vi "time_sub_frame.vi"(7 "Case select":string, 8 "felharmonikus N":i32=2, 9 "SNR window width [Hz]":dbl=0.4 format="%#_13g", 11 "path to binary file":path) -> (3 "output cluster":T1)   [LabVIEW 2017]
uses:
  <vilib>/Utility/file.llb/Read Delimited Spreadsheet (string).vi
  <vilib>/regexp/Match Regular Expression.xnode
panel:
  out "Array 2":dbl[](array[numeric])
  out "header":T2
  out "impulse szum/time (bigger better)":cluster{"X":dbl, "Y":dbl}[](graph)
  out "X SNR 3 (bigger better)":cluster{"X":dbl, "Y":dbl}[](graph)
  out "X SNR 4":cluster{"X":dbl, "Y":dbl}[](graph)
  out "X SNR":cluster{"X":dbl, "Y":dbl}[](graph)
  out "impulse mean (?)":cluster{"X":dbl, "Y":dbl}[](graph)
  out "impulse sd (?)":cluster{"X":dbl, "Y":dbl}[](graph)
  out "impulse szum (?)":cluster{"X":dbl, "Y":dbl}[](graph)
  out "enable":bool
  out "end":timestamp
  out "start":timestamp
  out "state":string
  out "saved":string
  out "all rows":string[][](array[string])
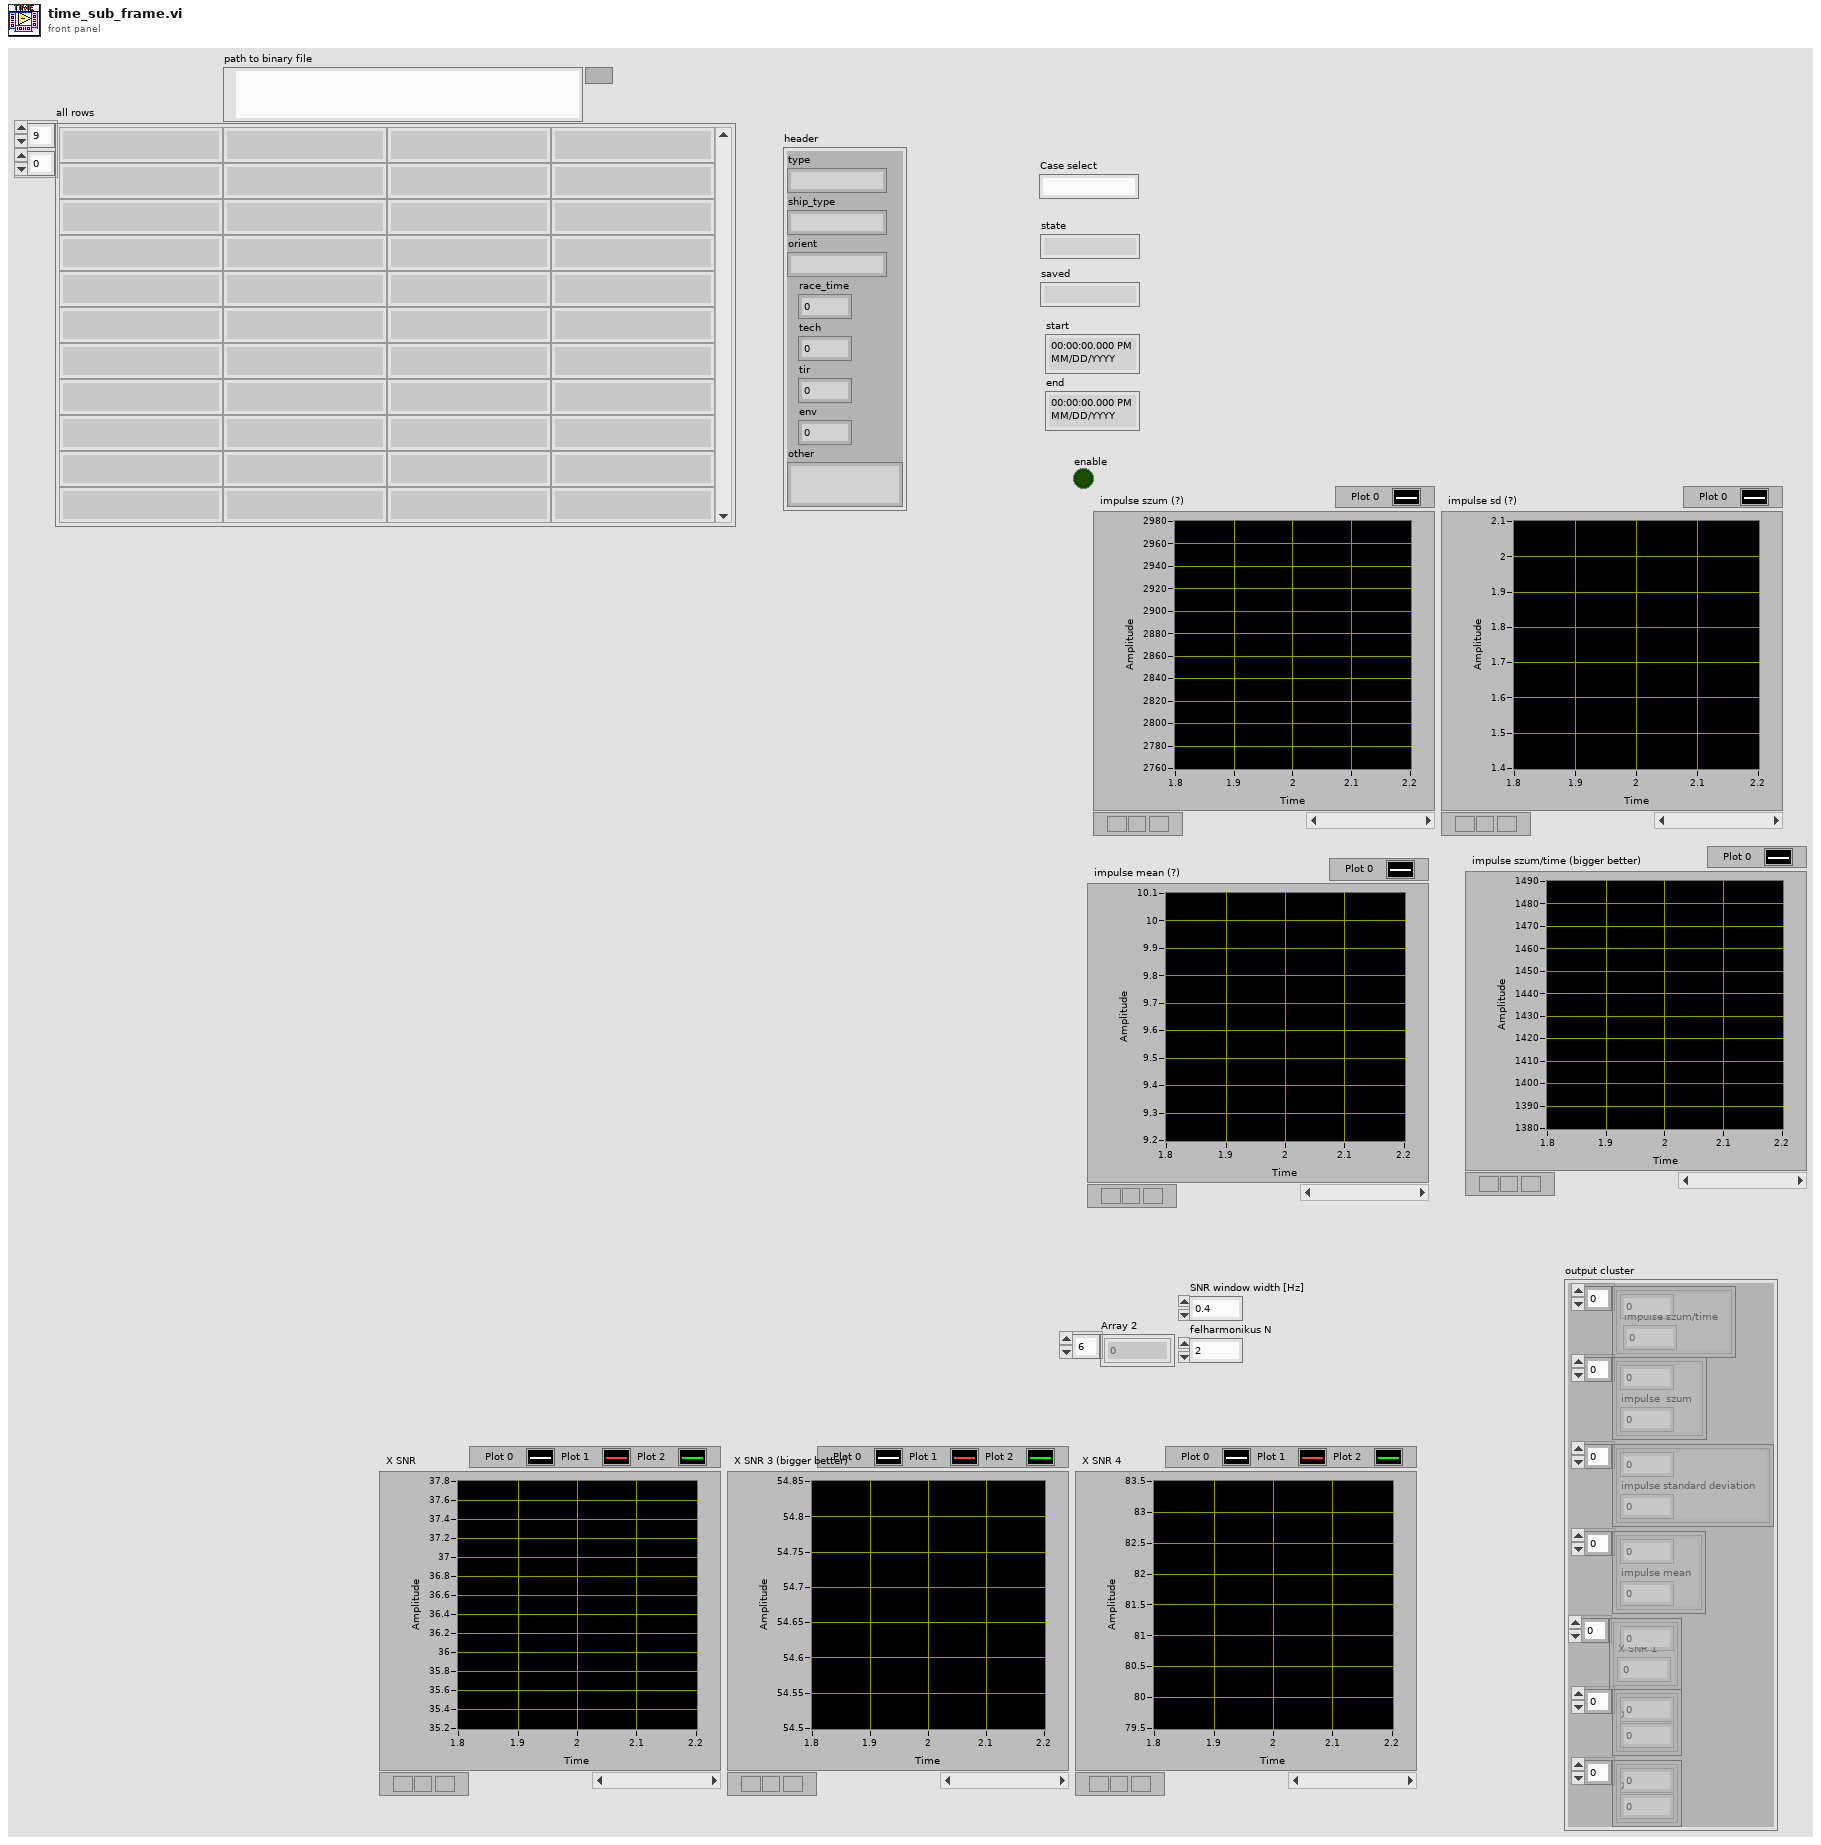
[diagram p1: front panel]
types:
  T1 = cluster{cluster{dbl, "impulse szum/time":dbl}[], cluster{dbl, "impulse  szum":dbl}[], cluster{dbl, "impulse standard deviation":dbl}[], cluster{dbl, "impulse mean":dbl}[], cluster{dbl, "X SNR 1":dbl}[], cluster{dbl, "X SNR 2":dbl}[], cluster{dbl, "X SNR 3":dbl}[]}
  T2 = cluster{"type":string, "ship_type":string, "orient":string, "race_time":dbl, "tech":dbl, "tir":dbl, "env":dbl, "other":string}
  T3 = cluster{cluster{dbl, "impulse szum/time":dbl}[], cluster{dbl, "impulse  szum":dbl}[], cluster{dbl, "impulse standard deviation":dbl}[], cluster{dbl, "impulse mean":dbl}[], cluster{dbl, dbl}[], cluster{dbl, dbl}[], cluster{dbl, dbl}[]}
  T4 = cluster{"path to binary file":path, "Start Cursor":timestamp, "Sec":dbl, "crossing level":dbl, "threshold":dbl, "avg window size":i32, "peak detect width":i32, "invert":bool, "SNR window width [Hz]":dbl, "felharmonikus N":i32, "End cursor":timestamp}
  T5 = cluster{"Átlag Csapásszám [stroke/m]":dbl, "mean of peaks":dbl, "impulse standard deviation":dbl, "impulse  szum":dbl, "standard deviation of peaks":dbl, "impulse mean":dbl, "X axis SNR mean":dbl, "X axis SNR standard deviation":dbl, "Y axis SNR standard deviation":dbl, "Y axis SNR mean":dbl, "resultant SNR standard deviation":dbl, "resultant SNR mean":dbl, "Z axis SNR standard deviation":dbl, "Z axis SNR mean":dbl, "impulse szum/mean":dbl}
  T6 = cluster{cluster{dbl, dbl}[], cluster{dbl, "impulse  szum":dbl}[], cluster{dbl, "impulse standard deviation":dbl}[], cluster{dbl, "impulse mean":dbl}[], cluster{dbl, dbl}[], cluster{dbl, dbl}[], cluster{dbl, dbl}[]}
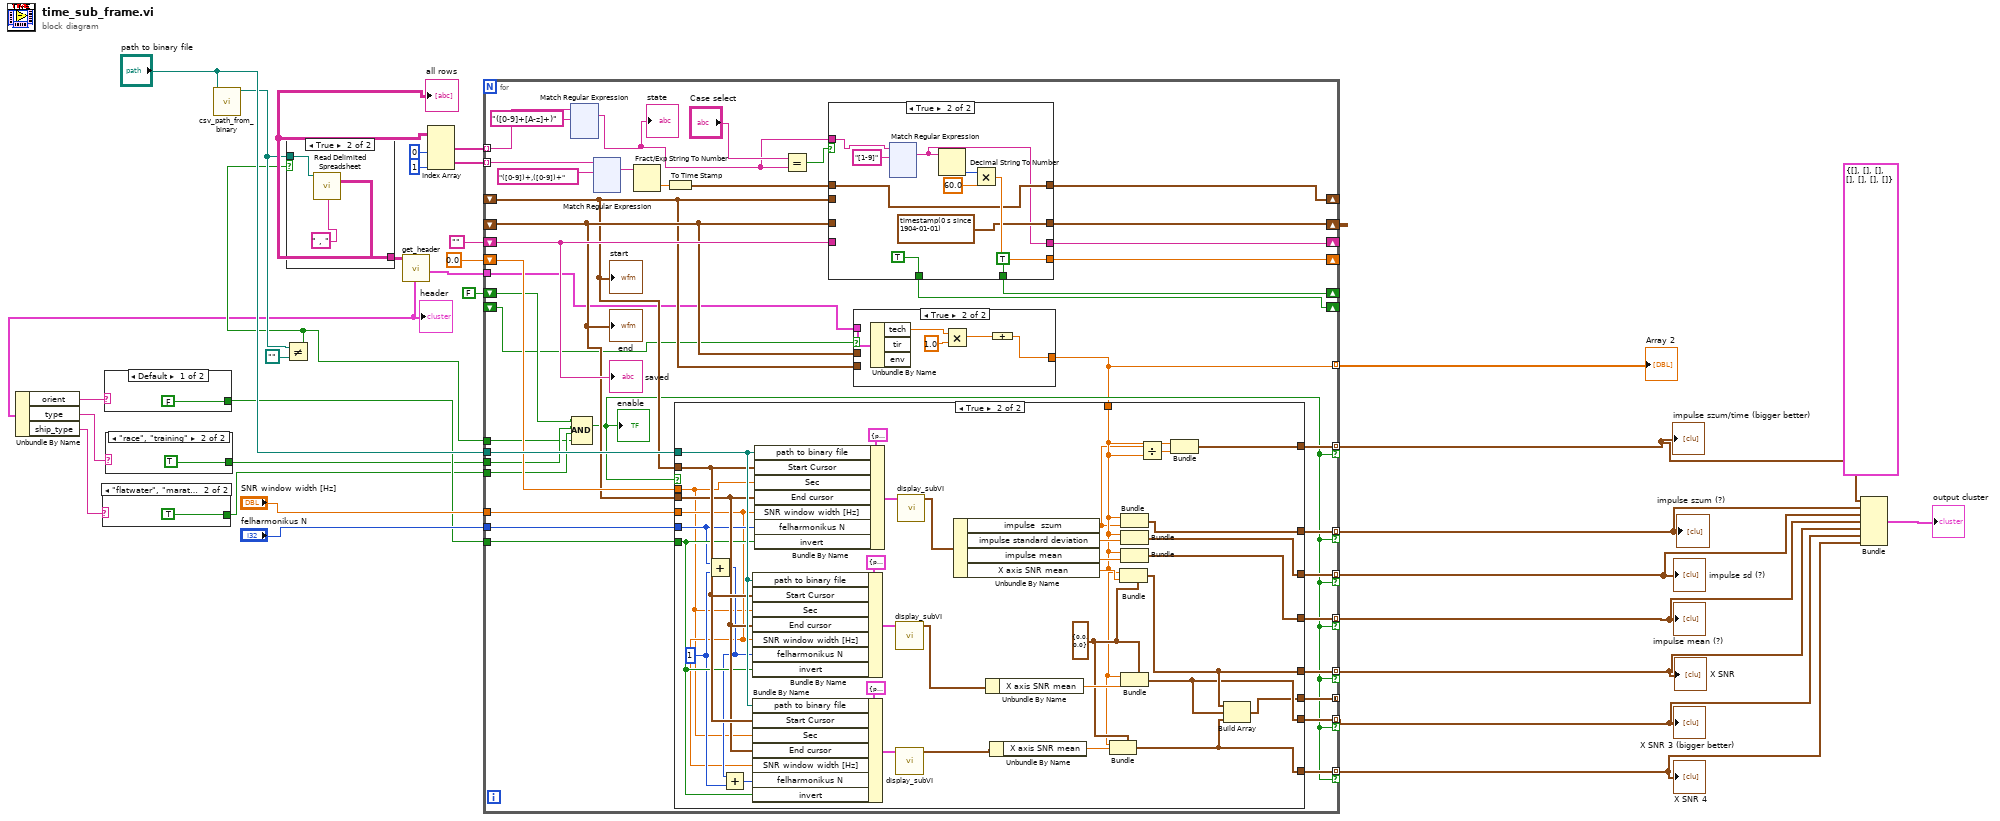
[diagram p0: block diagram]
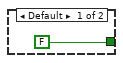
[diagram p3: hidden frame]
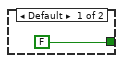
[diagram p4: hidden frame]
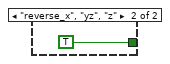
[diagram p5: hidden frame]
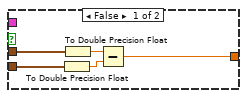
[diagram p6: hidden frame]
diagram:
  (unwired) T3 {[], [], [], [], [], [], []} ("output cluster")
  n1 = call "csv_path_from_binary.vi"("path to binary file"="path to binary file") -> ("path to spec. ext."=w5:path)  [unwired: 10 in]
  n2 = Not Equal?(x=w5, y=path "") -> (x != y?=w4:bool)
  n3 = case shown="True" w4 {
    tunnel: [_ w32] -> w6
    tunnel: w5 -> [_ w31]
    frame False {
    }
    frame True {
      n4 = call-poly <vilib>:"Read Delimited Spreadsheet.vi"("file path (dialog if empty)"=w31, "delimiter (\\t)"=" , " ("delimiter (\\t)")) -> ("all rows"=w32:string[][])  [unwired: 8 in, 5 out]
    }
  }
  "all rows" <- w6
  n5 = call "get_header.vi"("all rows"=w6) -> ("header"=w2:T2)  [unwired: 10 in]
  "header" <- w2
  n6 = Unbundle By Name(w2) -> ("orient"=w21:string, "type"=w11:string, "ship_type"=w9:string)
  n7 = case shown="\"flatwater\", \"marathon\"" w9 {
    tunnel: [FALSE TRUE] -> w8
    frame Default {
    }
    frame "flatwater", "marathon" {
    }
  }
  n8 = case shown="Default" w21 {
    tunnel: [FALSE TRUE] -> w20
    frame Default {
    }
    frame "reverse_x", "yz", "z" {
    }
  }
  n9 = case shown="\"race\", \"training\"" w11 {
    tunnel: [FALSE TRUE] -> w10
    frame Default {
    }
    frame "race", "training" {
    }
  }
  n10 = Index Array(array=w6, index (col) #1=0 ("disabled index (col)"), index (col) #2=1 ("index (col)")) -> (element #1=w29:string[], element #2=w30:string[])  [unwired: 2 in]
  n11 = for {
    tunnel: w30 -> [w76] mode=indexing
    tunnel: w29 -> [w71] mode=indexing
    shift-right: [w74] -> _
    shift-left: _ -> [w61]
    shift-right: [w73] -> _
    shift-left: _ -> [w62]
    shift-right: [w72] -> _
    shift-left: "" -> [w69]
    shift-right: [w47] -> _
    shift-left: 0.0 ("Sec") -> [w66]
    shift-right: [w68] -> _
    shift-left: FALSE -> [w51]
    tunnel: "path to binary file" -> [w67]
    tunnel: "SNR window width [Hz]" -> [w65]
    tunnel: "felharmonikus N" -> [w64]
    tunnel: w20 -> [w63]
    tunnel: [w60] -> w18 mode=indexing if=w52
    tunnel: [w59] -> w17 mode=indexing if=w52
    tunnel: [w58] -> w16 mode=indexing if=w52
    tunnel: [w57] -> w15 mode=indexing if=w52
    tunnel: [w56] -> w14 mode=indexing if=w52
    tunnel: [w55] -> w13 mode=indexing if=w52
    tunnel: [w54] -> _ mode=concatenating
    tunnel: [w53] -> w19 mode=indexing if=w52
    tunnel: w10 -> [w50]
    tunnel: w8 -> [w49]
    tunnel: w4 -> [w48]
    tunnel: w2 -> [w46]
    tunnel: [w45] -> w1 mode=indexing
    shift-right: [w44] -> _
    shift-left: _ -> [w43]
    n12 = xnode "Match Regular Expression"("input string"=w71, "regular expression"="([0-9]+[A-z]+)") -> ("whole match"=w41:string)  [unwired: 4 in, 4 out]
    "state" <- w41
    n13 = Compound Arithmetic op=AND(w51, w50, w49, w48) -> (w52:bool)
    "enable" <- w52
    n14 = xnode "Match Regular Expression"("input string"=w76, "regular expression"="([0-9])+,([0-9])+") -> ("whole match"=w78:string)  [unwired: 4 in, 4 out]
    n15 = Fract/Exp String To Number(string=w78) -> (number=w77:dbl)  [unwired: 3 in, 1 out]
    n16 = To Time Stamp(1:w77) -> (0:w75:timestamp)
    n17 = Equal?(x="Case select", y=w41) -> (x = y?=w40:bool)
    n18 = case shown="True" w40 {
      tunnel: [w240 w248] -> w74
      tunnel: w75 -> [_ w248]
      tunnel: [w241 timestamp(0 s since 1904-01-01) ("f")] -> w73
      tunnel: [w242 w244] -> w72
      tunnel: w69 -> [w242 _]
      tunnel: [_ w249] -> w47
      tunnel: w62 -> [w241 _]
      tunnel: w61 -> [w240 _]
      tunnel: [_ TRUE] -> w68
      tunnel: [_ TRUE] -> w44
      tunnel: w41 -> [_ w243]
      frame False {
      }
      frame True {
        n19 = xnode "Match Regular Expression"("input string"=w243, "regular expression"="[1-9]") -> ("whole match"=w244:string)  [unwired: 4 in, 4 out]
        n20 = Decimal String To Number(string=w244) -> (number=w250:i32)  [unwired: 2 in, 1 out]
        n21 = Multiply(x=w250, y=60.0) -> (x*y=w249:dbl)
      }
    }
    n22 = case shown="True" w43 {
      tunnel: w62 -> [w84 _]
      tunnel: w61 -> [w83 _]
      tunnel: [w80 w86] -> w45
      tunnel: w46 -> [_ w89]
      frame False {
        n23 = To Double Precision Float(number=w83) -> (double precision float=w81:dbl)
        n24 = To Double Precision Float(number=w84) -> (double precision float=w82:dbl)
        n25 = Subtract(x=w82, y=w81) -> (x-y=w80:dbl)
      }
      frame True {
        n26 = Unbundle By Name(w89) -> ("tech"=w88:dbl)  [unwired: 2 out]
        n27 = Multiply(x=w88, y=1.0) -> (x*y=w85:dbl)
        n28 = Compound Arithmetic op=ADD(w85) -> (w86:dbl)
      }
    }
    n29 = case shown="True" w52 {
      tunnel: w67 -> [_ w119]
      tunnel: w61 -> [_ w118]
      tunnel: w62 -> [_ w117]
      tunnel: w66 -> [_ w110]
      tunnel: w65 -> [_ w111]
      tunnel: w64 -> [_ w115]
      tunnel: w63 -> [_ w116]
      tunnel: w45 -> [_ w91]
      tunnel: [_ w105] -> w60
      tunnel: [_ w104] -> w59
      tunnel: [_ w103] -> w58
      tunnel: [_ w98] -> w57
      tunnel: [_ w97] -> w56
      tunnel: [_ w96] -> w55
      tunnel: [_ w95] -> w54
      tunnel: [_ w93] -> w53
      frame False {
      }
      frame True {
        w94 = cluster{dbl, dbl} {0.0, 0.0} ("cluster")
        w112 = 1
        n30 = Add(x=w115, y=w112) -> (x+y=w113:i32)
        n31 = Add(x=w113, y=w112) -> (x+y=w114:i32)
        n32 = Bundle By Name(cluster=T4 {"path to binary file"=path "C:/Users/Lenovo/Desktop/szakdoga/data", "Start Cursor"=timestamp(0 s since 1904-01-01), "Sec"=60.0, "crossing level"=0.0, "threshold"=0.35, "avg window size"=5, "peak detect width"=30, "invert"=FALSE, "SNR window width [Hz]"=0.5, "felharmonikus N"=2, "End cursor"=timestamp(0 s since 1904-01-01)} ("input cluster"), "path to binary file"=w119, "Start Cursor"=w118, "Sec"=w110, "End cursor"=w117, "SNR window width [Hz]"=w111, "felharmonikus N"=w113, "invert"=w116) -> (w122:T4)
        n33 = Bundle By Name(cluster=T4 {"path to binary file"=path "C:/Users/Lenovo/Desktop/szakdoga/data", "Start Cursor"=timestamp(0 s since 1904-01-01), "Sec"=60.0, "crossing level"=0.0, "threshold"=0.35, "avg window size"=5, "peak detect width"=30, "invert"=FALSE, "SNR window width [Hz]"=0.5, "felharmonikus N"=2, "End cursor"=timestamp(0 s since 1904-01-01)} ("input cluster"), "path to binary file"=w119, "Start Cursor"=w118, "Sec"=w110, "End cursor"=w117, "SNR window width [Hz]"=w111, "felharmonikus N"=w114, "invert"=w116) -> (w121:T4)
        n34 = Bundle By Name(cluster=T4 {"path to binary file"=path "C:/Users/Lenovo/Desktop/szakdoga/data", "Start Cursor"=timestamp(0 s since 1904-01-01), "Sec"=60.0, "crossing level"=0.0, "threshold"=0.35, "avg window size"=5, "peak detect width"=30, "invert"=FALSE, "SNR window width [Hz]"=0.5, "felharmonikus N"=2, "End cursor"=timestamp(0 s since 1904-01-01)} ("input cluster"), "path to binary file"=w119, "Start Cursor"=w118, "Sec"=w110, "End cursor"=w117, "SNR window width [Hz]"=w111, "felharmonikus N"=w115, "invert"=w116) -> (w125:T4)
        n35 = call "display_subVI.vi"("input cluster"=w122) -> ("data cluster"=w107:T5)  [unwired: 10 in]
        n36 = call "display_subVI.vi"("input cluster"=w121) -> ("data cluster"=w99:T5)  [unwired: 10 in]
        n37 = call "display_subVI.vi"("input cluster"=w125) -> ("data cluster"=w106:T5)  [unwired: 10 in]
        n38 = Unbundle By Name(w106) -> ("impulse  szum"=w90:dbl, "impulse standard deviation"=w108:dbl, "impulse mean"=w109:dbl, "X axis SNR mean"=w102:dbl)
        n39 = Unbundle By Name(w107) -> ("X axis SNR mean"=w101:dbl)
        n40 = Unbundle By Name(w99) -> ("X axis SNR mean"=w100:dbl)
        n41 = Bundle(cluster=w94, w91, w100) -> (w96:cluster{dbl, dbl})
        n42 = Bundle(cluster=w94, w91, w102) -> (w98:cluster{dbl, dbl})
        n43 = Bundle(w91, "impulse  szum"=w90) -> (w105:cluster{dbl, "impulse  szum":dbl})  [unwired: 1 in]
        n44 = Bundle(w91, "impulse standard deviation"=w108) -> (w104:cluster{dbl, "impulse standard deviation":dbl})  [unwired: 1 in]
        n45 = Bundle(w91, "impulse mean"=w109) -> (w103:cluster{dbl, "impulse mean":dbl})  [unwired: 1 in]
        n46 = Bundle(cluster=w94, w91, w101) -> (w97:cluster{dbl, dbl})
        n47 = Divide(x=w90, y=w91) -> (x/y=w92:dbl)
        n48 = Bundle(w91, w92) -> (w93:cluster{dbl, dbl})  [unwired: 1 in]
        n49 = Build Array(w98, w97, w96) -> (w95:cluster{dbl, dbl}[])
      }
    }
    "saved" <- w69
    "start" <- w61
    "end" <- w62
  }
  "impulse szum (?)" <- w18
  "impulse sd (?)" <- w17
  "impulse mean (?)" <- w16
  "X SNR" <- w15
  "X SNR 4" <- w13
  "X SNR 3 (bigger better)" <- w14
  "impulse szum/time (bigger better)" <- w19
  "Array 2" <- w1
  n50 = Bundle(w19, w18, w17, w16, w15, w14, w13) -> (→"output cluster":T6)  [unwired: 1 in]
